vi "Read Actor Name.vi"(8 "error in (no error)":errorcluster, 11 "Generic Actor in":refnum<class "Generic Actor.lvclass">) -> (0 "error out":errorcluster, 2 "Actor Name":string, 3 "Generic Actor out":refnum<class "Generic Actor.lvclass">)   [LabVIEW 2020, in "Generic Actor.lvlib" / "Generic Actor.lvclass"]
uses:
  Generic Actor.lvclass
  Generic Actor.lvclass/Generic Actor.ctl
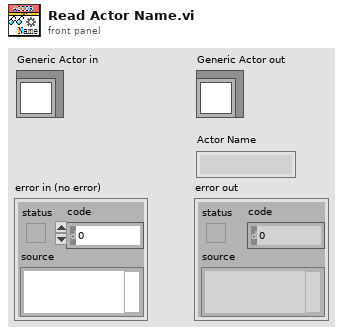
[diagram p1: front panel]
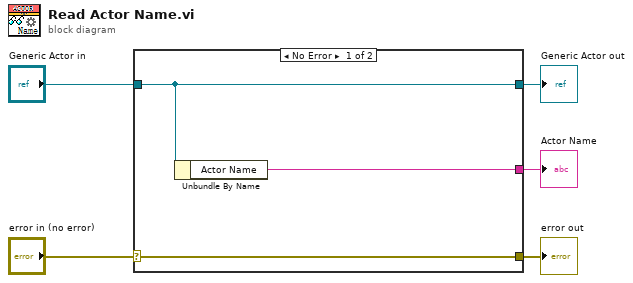
[diagram p0: block diagram]
diagram:
  n1 = case shown="No Error" "error in (no error)" {
    selector: "error in (no error)" -> [w8 w9]
    tunnel: [w8 w9] -> w4
    tunnel: [w7 w10] -> w2
    tunnel: "Generic Actor in" -> [w7 w10]
    tunnel: [w6 _] -> w1
    frame No Error {
      n2 = Unbundle By Name(w7) -> ("Actor Name"=w6:string)
    }
    frame Error {
    }
  }
  "error out" <- w4
  "Generic Actor out" <- w2
  "Actor Name" <- w1
